vi "tsfifo_add_lin_pass_filter.vi"(8 "错误输入（无错误）":errorcluster, 9 "AIdentifier":i32, 10 "AChn":i32, 11 "路径输入":path) -> (0 "错误输出":errorcluster, 2 "return":i32, 3 "路径输出":path)   [LabVIEW 2014]
doc: "Function Introduction :\nAdd Lin message through filter\nCall location :\ninput parameter :\nAChn: Channel\nAIdentifier: Message ID\nReturn value :\n==0: Execution successful\nOther values: Query error code"
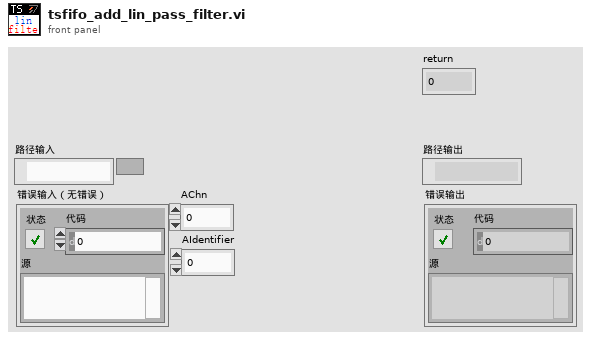
[diagram p1: front panel]
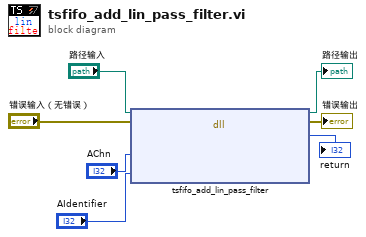
[diagram p0: block diagram]
diagram:
  n1 = dll-call lib="D:/Program Files (x86)/TOSUN/TSMaster/Data/SDK/lib/x86/TSMaster.dll" fn="tsfifo_add_lin_pass_filter"(path in="路径输入", error in="错误输入（无错误）", "AChn"="AChn", "AIdentifier"="AIdentifier") -> (path out=→"路径输出":path, error out=→"错误输出":errorcluster, "返回类型"=→"return":i32)  [unwired: 3 in]
